vi "WSVCAP SHL Host TL I2C Read - Multiple Device.vi"(0 "Bytes to Read (1-4)":u8=4 min=1 max=4 step=1, 5 "Sub Address [U8]":u8=191 format="%.0x", 11 "error in":errorcluster, 13 "Log (T)":bool=TRUE, 14 "FPGA":T1) -> (4 "C1:1-36 Read Data [U8]":u8[][](array[numeric]) format="%.0x", 6 "C2:1-36 Read Data [U8]":u8[][](array[numeric]) format="%.0x", 8 "C3:1-36 Read Data [U8]":u8[][](array[numeric]) format="%.0x", 15 "error out":errorcluster)   [LabVIEW 2012]
uses:
  Type Defs/WSVCAP SHL I2C FPGA Enum.ctl
panel:
  in  "DUT Mask Array (All)":bool[][](array[boolean])=[[TRUE, TRUE, TRUE, TRUE, TRUE, TRUE, TRUE, TRUE, TRUE, TRUE, TRUE, TRUE, TRUE, TRUE, TRUE, TRUE, TRUE, TRUE, TRUE, TRUE, TRUE, TRUE, TRUE, TRUE, TRUE, TRUE, TRUE, TRUE, TRUE, TRUE, TRUE, TRUE, TRUE, TRUE, TRUE, TRUE], [TRUE, TRUE, TRUE, TRUE, TRUE, TRUE, TRUE, TRUE, TRUE, TRUE, TRUE, TRUE, TRUE, TRUE, TRUE, TRUE, TRUE, TRUE, TRUE, TRUE, TRUE, TRUE, TRUE, TRUE, TRUE, TRUE, TRUE, TRUE, TRUE, TRUE, TRUE, TRUE, TRUE, TRUE, TRUE, TRUE], [TRUE, TRUE, TRUE, TRUE, TRUE, TRUE, TRUE, TRUE, TRUE, TRUE, TRUE, TRUE, TRUE, TRUE, TRUE, TRUE, TRUE, TRUE, TRUE, TRUE, TRUE, TRUE, TRUE, TRUE, TRUE, TRUE, TRUE, TRUE, TRUE, TRUE, TRUE, TRUE, TRUE, TRUE, TRUE, TRUE], [FALSE, FALSE, FALSE, FALSE, FALSE, FALSE, FALSE, FALSE, FALSE, FALSE, FALSE, FALSE, FALSE, FALSE, FALSE, FALSE, TRUE, FALSE, FALSE, FALSE, FALSE, FALSE, TRUE, FALSE, FALSE, FALSE, FALSE, FALSE, FALSE, FALSE, FALSE, TRUE, FALSE, FALSE, FALSE, FALSE]]
  out "Socket Mask Set [U64]":u64[](array[numeric]) format="%012x"
  out "Data Headers":u8[](array[numeric])=[1, 2, 3, 4, 5, 6, 7, 8, 9, 10, 11, 12, 12, 14, 15, 16, 17, 18, 19, 20, 21, 22, 23, 24, 25, 26, 27, 28, 29, 30, 31, 32, 33, 34, 35, 36]
  # "DUT 01"
  # "DUT 02"
  # "DUT 03"
  # "DUT 04"
  # "DUT 05"
  # "DUT 06"
  # "DUT 07"
  # "DUT 08"
  # "DUT 09"
  # "DUT 10"
  # "DUT 11"
  # "DUT 12"
  # "DUT 13"
  # "DUT 14"
  # "DUT 15"
  # "DUT 16"
  # "DUT 17"
  # "DUT 18"
  # "DUT 19"
  # "DUT 20"
  # "DUT 21"
  # "DUT 22"
  # "DUT 23"
  # "DUT 24"
  # "DUT 25"
  # "DUT 26"
  # "DUT 27"
  # "DUT 28"
  # "DUT 29"
  # "DUT 30"
  # "DUT 31"
  # "DUT 32"
  # "DUT 33"
  # "DUT 34"
  # "DUT 35"
  # "DUT 36"
  # "C1"
  # "C2"
  # "C3"
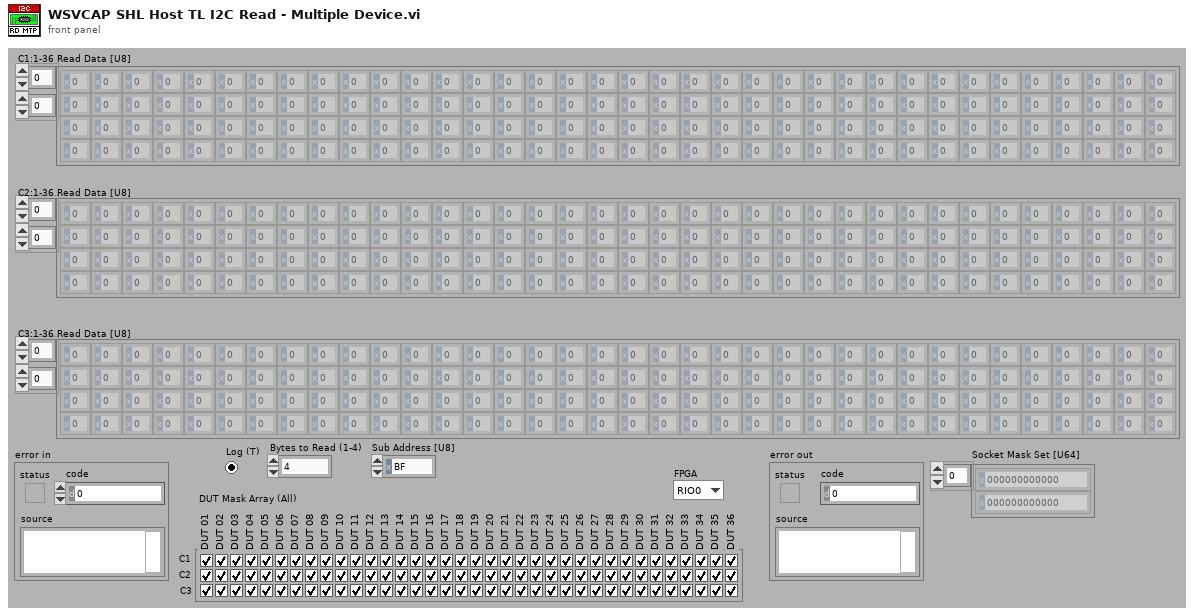
[diagram p1: front panel]
types:
  T1 = typedef "WSVCAP SHL I2C FPGA Enum.ctl" = enum16{"RIO0", "RIO1"}
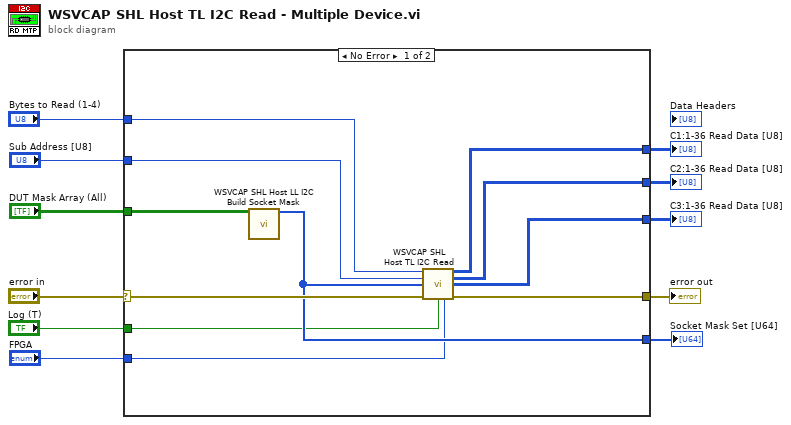
[diagram p0: block diagram]
diagram:
  n1 = case shown="No Error" "error in" {
    selector: "error in" -> [w21 w23]
    tunnel: [w22 w23] -> w11
    tunnel: "Bytes to Read (1-4)" -> [w20 _]
    tunnel: "Sub Address [U8]" -> [w19 _]
    tunnel: [w16 _] -> w7
    tunnel: [w18 _] -> w6
    tunnel: [w17 _] -> w5
    tunnel: "DUT Mask Array (All)" -> [w15 _]
    tunnel: "Log (T)" -> [w14 _]
    tunnel: [w13 _] -> w2
    tunnel: "FPGA" -> [w12 _]
    frame No Error {
      n2 = call "WSVCAP SHL Host LL I2C Build Socket Mask.vi"("DUT Mask Array"=w15) -> ("Socket Mask Set [U64]"=w16:u64[])  [unwired: 14 in]
      n3 = call "WSVCAP SHL Host TL I2C Read.vi"("Bytes to Read"=w20, "Sub Address [U8]"=w19, "Socket Mask Set [U64]"=w16, "error in"=w21, "Log (T)"=w14, "FPGA"=w12) -> ("C1 Read Data Out"=w18:u8[][], "C2 Read Data Out"=w17:u8[][], "C3 Read Data Out"=w13:u8[][], "error out"=w22:errorcluster)  [unwired: 6 in]
    }
    frame Error {
    }
  }
  "error out" <- w11
  "Socket Mask Set [U64]" <- w7
  "C1:1-36 Read Data [U8]" <- w6
  "C2:1-36 Read Data [U8]" <- w5
  "C3:1-36 Read Data [U8]" <- w2
